vi "并行循环.vi"() -> ()   [LabVIEW 2015]
panel:
  in  "停止":bool
  in  "暂停采集":bool
  out "波形图表 2":dbl(graph)
  out "波形图表":dbl(graph)
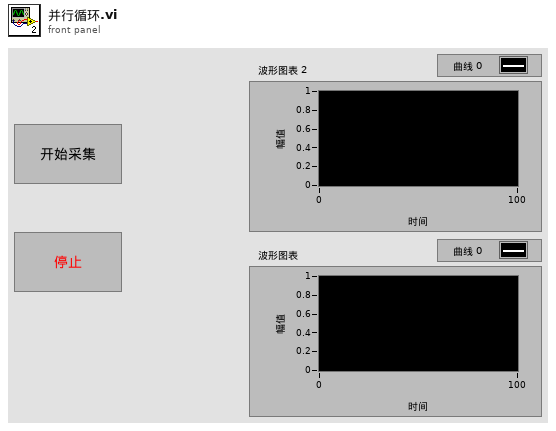
[diagram p1: front panel]
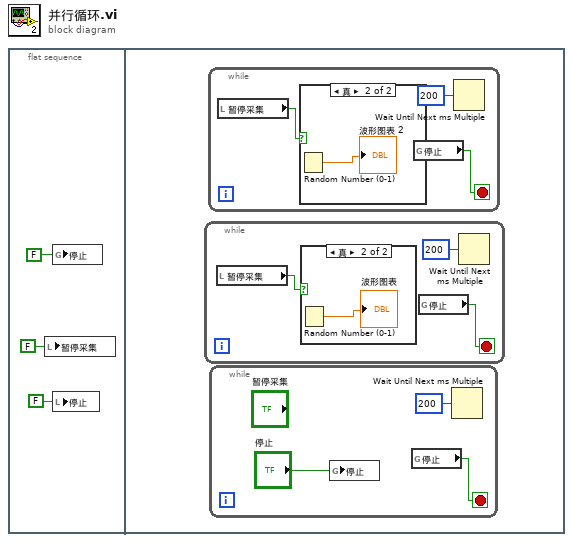
[diagram p0: block diagram]
diagram:
  n1 = flat-sequence {
    frame #0 {
      n2 = local write "暂停采集"(FALSE ("暂停采集")) -> ()
      n3 = global write "全局 1.vi" "停止"(FALSE ("停止")) -> ()
      n4 = local write "停止"(FALSE ("停止")) -> ()
    }
    frame #1 {
      n5 = while {
        stop <- w13 stop-if-true
        n6 = local read "暂停采集"() -> (w11:bool)
        n7 = case shown="真" w11 {
          frame False {
          }
          frame True {
            n8 = Random Number (0-1)() -> (number: 0 to 1=→"波形图表":dbl)
          }
        }
        n9 = global read "全局 1.vi" "停止"() -> (w13:bool)
        n10 = Wait Until Next ms Multiple(millisecond multiple=u32 200 ("毫秒倍数")) -> ()  [unwired: 1 out]
      }
      n11 = while {
        stop <- w9 stop-if-true
        n12 = local read "暂停采集"() -> (w7:bool)
        n13 = case shown="真" w7 {
          frame False {
          }
          frame True {
            n14 = Random Number (0-1)() -> (number: 0 to 1=→"波形图表 2":dbl)
          }
        }
        n15 = global read "全局 1.vi" "停止"() -> (w9:bool)
        n16 = Wait Until Next ms Multiple(millisecond multiple=u32 200 ("毫秒倍数")) -> ()  [unwired: 1 out]
      }
      n17 = while {
        stop <- w6 stop-if-true
        n18 = global write "全局 1.vi" "停止"("停止") -> ()
        n19 = global read "全局 1.vi" "停止"() -> (w6:bool)
        n20 = Wait Until Next ms Multiple(millisecond multiple=u32 200 ("毫秒倍数")) -> ()  [unwired: 1 out]
      }
    }
  }
